vi "showMessage.vi"(8 "error in (no error)":errorcluster, 9 "Message":string, 10 "User.lvclass":refnum<class "User.lvclass">, 11 "ChatRoom in":refnum<class "ChatRoom.lvclass">) -> (0 "error out":errorcluster, 3 "ChatRoom out":refnum<class "ChatRoom.lvclass">)   [LabVIEW 2018, in "ChatRoom.lvclass"]
uses:
  ChatRoom.lvclass
  User Class/User.lvclass
  ConsoleOut/Print Options.ctl
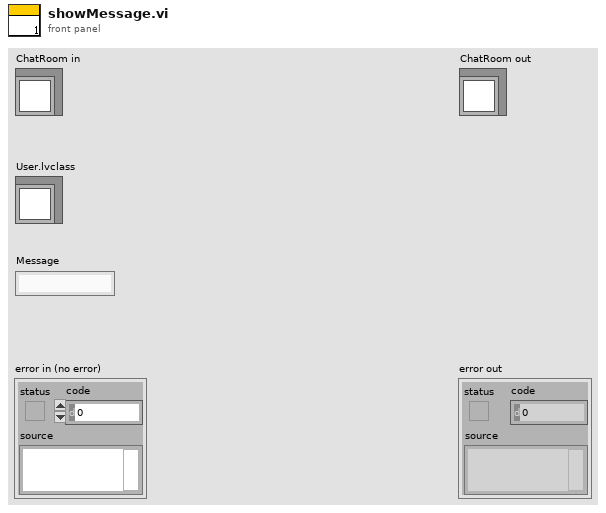
[diagram p1: front panel]
types:
  T1 = typedef "Print Options.ctl" = enum16{"Create", "Get Reference", "Print", "Print Header", "Close"}
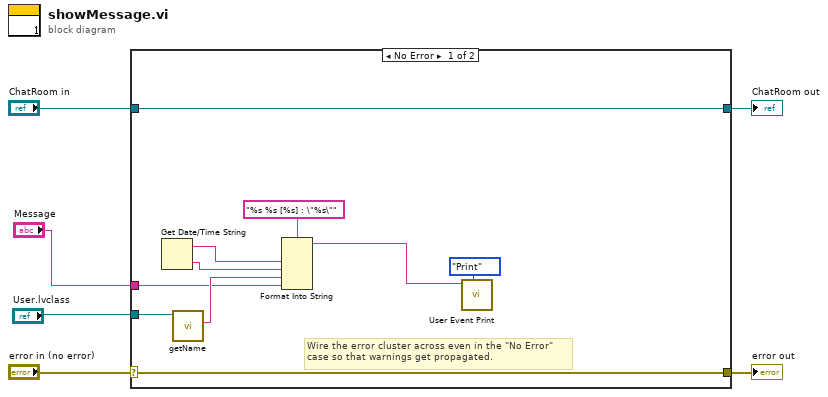
[diagram p0: block diagram]
diagram:
  n1 = case shown="No Error" "error in (no error)" {
    selector: "error in (no error)" -> [w15 w18]
    tunnel: [w15 w18] -> w5
    tunnel: [w16 w17] -> w3
    tunnel: "ChatRoom in" -> [w16 w17]
    tunnel: "User.lvclass" -> [w12 _]
    tunnel: "Message" -> [w9 _]
    frame No Error {
      # "Wire the error cluster across even in the \"No Error\"\ncase so that warnings get propagated."
      n2 = Get Date/Time String() -> (date string=w14:string, time string=w13:string)  [unwired: 3 in]
      n3 = call-dynamic "getName.vi"("User in"=w12) -> ("name"=w10:string)  [unwired: 8 in, 2 out]
      n4 = Format Into String(format string="%s %s [%s] : \"%s\"", w14, w13, w10, w9) -> (resulting string=w8:string)  [unwired: 2 in, 1 out]
      n5 = call "User Event Print.vi"("Options"=Print_Options."Print", "String to Print"=w8) -> ()  [unwired: 8 in, 2 out]
    }
    frame Error {
    }
  }
  "error out" <- w5
  "ChatRoom out" <- w3
